vi "Main_UI.vi"(0 "Wait_Time (sec)":i32=2 caption="Wait Time (sec)" min=2, 5 "Exit":bool, 7 "Error_Log":bool caption="Error Log") -> (3 "BI_Error":T2 caption="Error?", 4 "Last_Read_PSRR (dB)":i32 caption="Last Read PSRR (dB)", 6 "Last_Error_Details":T1 caption="Last Error Details", 8 "Obtained_PSRR":i32(graph) caption="Obtained PSRR", 10 "Error_Log_Table":string[][](table) caption="Error Log Table")   [LabVIEW 2021]
doc: "This is the Main UI that Interact With the User"
uses:
  Controls/Update_Event.ctl
  Controls/Last_Error_Details.ctl
  Controls/BI_Error.ctl
panel:
  out "Error_Out":errorcluster
  in  "Error_In":errorcluster
  # "PSRR Monitor"
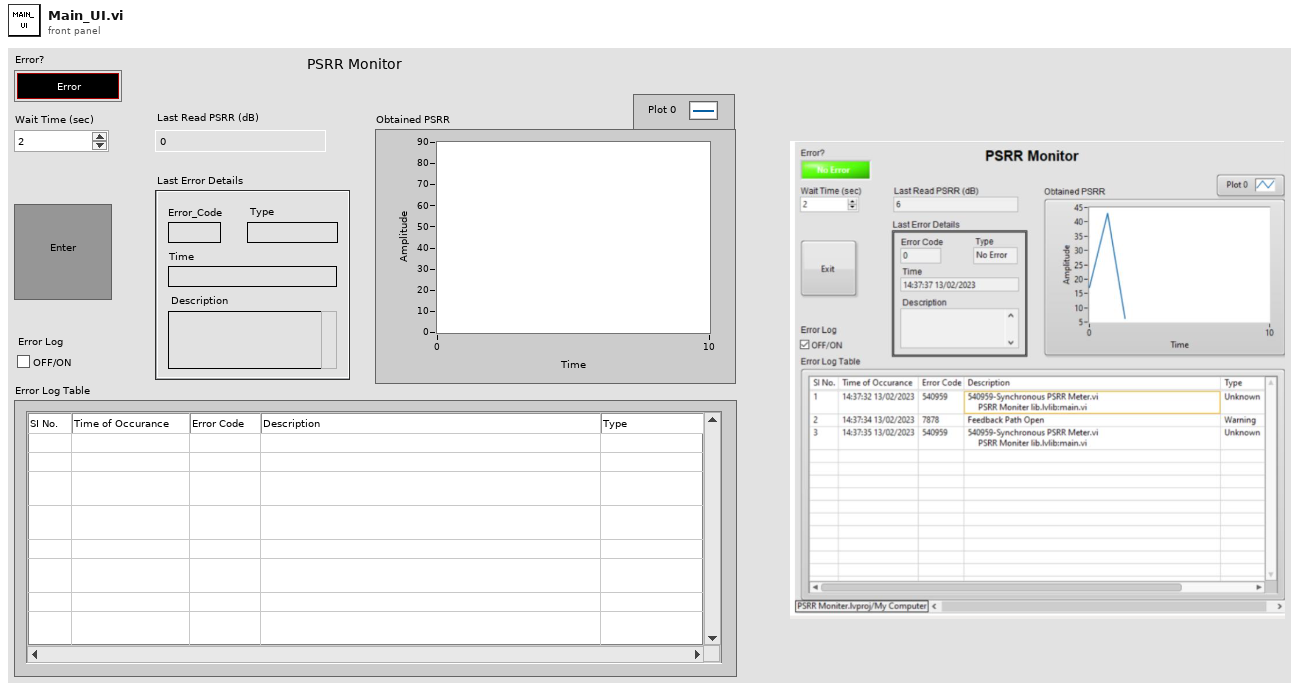
[diagram p1: front panel]
types:
  T1 = typedef "Last_Error_Details.ctl" = cluster{"Error_Code":string, "Type":string, "Time":string, "Description":string}
  T2 = typedef "BI_Error.ctl" = bool
  T3 = typedef "Update_Event.ctl" = cluster{"Exit":bool, "Wait_Time (sec)":i32}
  T4 = typedef "Obtained_PSRR_Data.ctl" = cluster{"Data":i32, "Obtained_PSRR_Data_Operation":T5}
  T5 = typedef "Obtained_PSRR_Data_Operation.ctl" = enum16{"Update", "Dont_Update", "Clear"}
  T6 = typedef "BI_Error_Con.ctl" = cluster{"Error?_Color":cluster{u32, u32}[], "Error?_Text":string}
  T7 = enum16{"Left Button", "Center Button", "Right Button", "Window Close"}
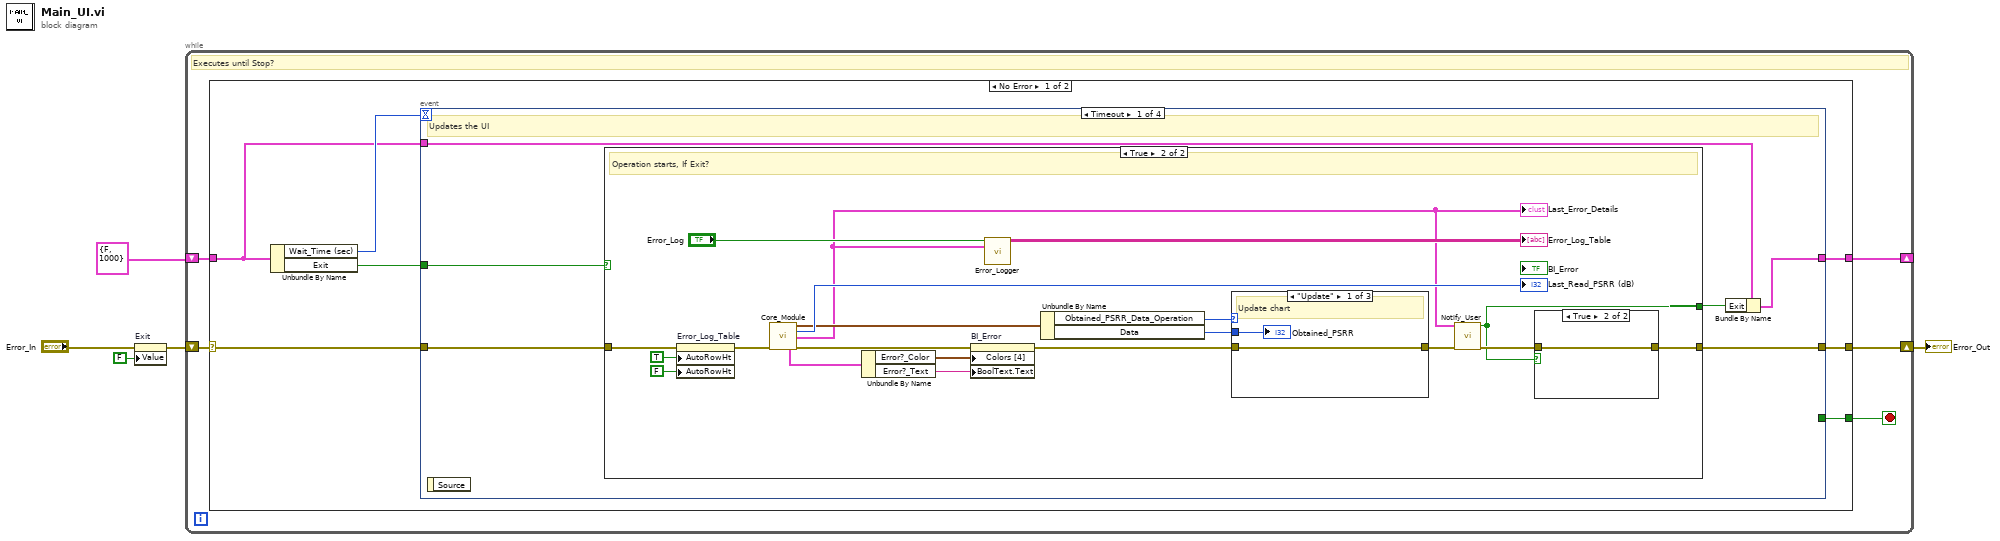
[diagram p0: block diagram]
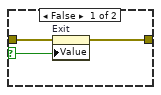
[diagram p3: hidden frame]
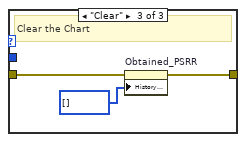
[diagram p5: hidden frame]
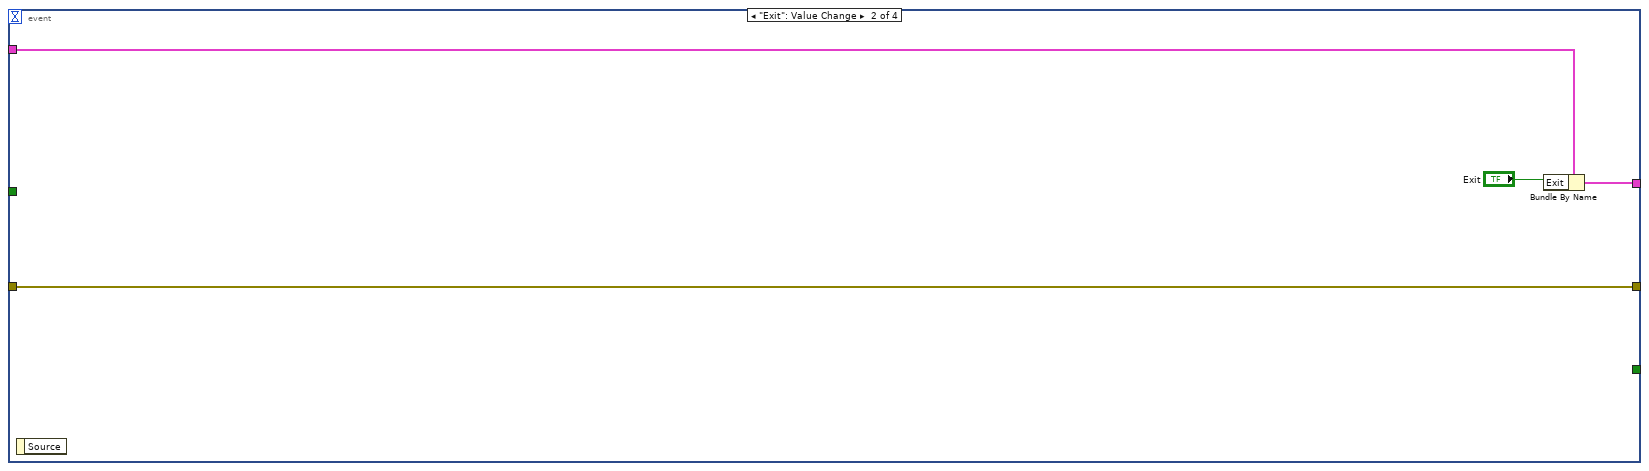
[diagram p6: hidden frame]
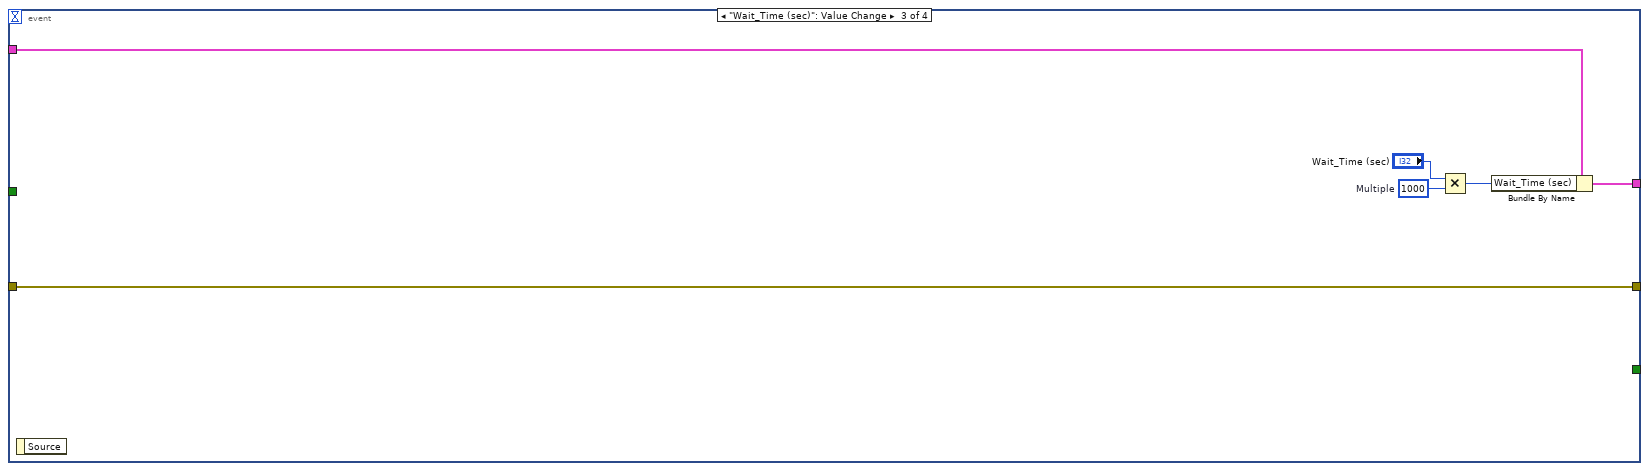
[diagram p7: hidden frame]
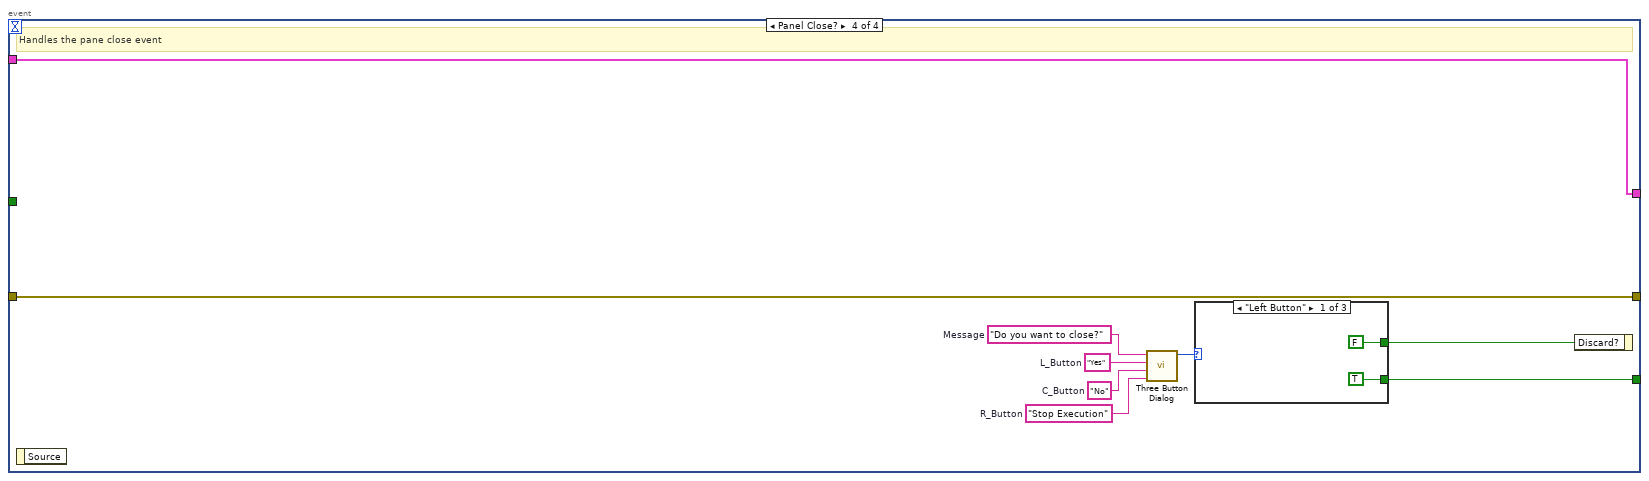
[diagram p8: hidden frame]
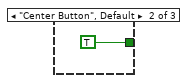
[diagram p9: hidden frame]
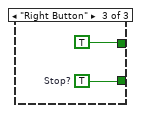
[diagram p10: hidden frame]
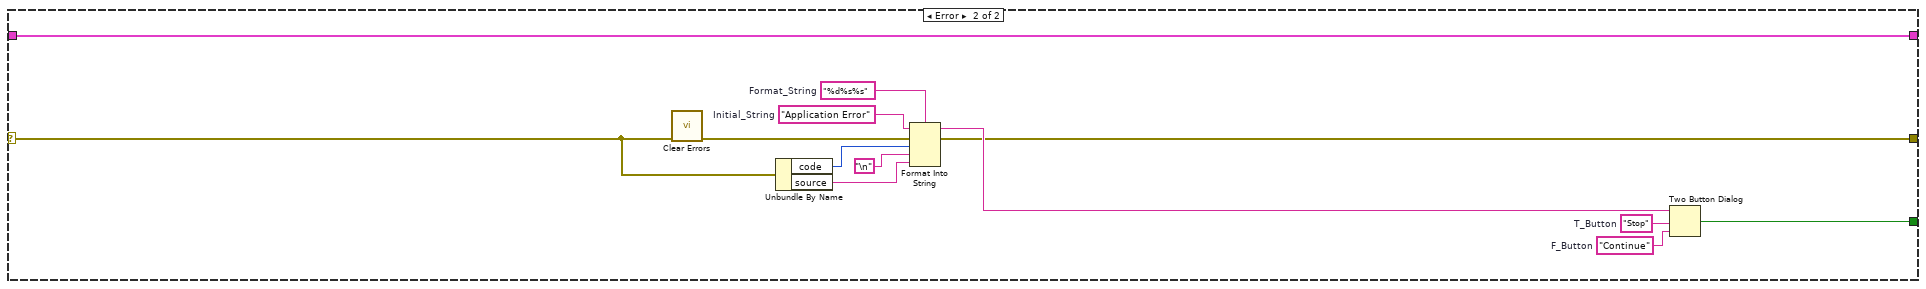
[diagram p11: hidden frame]
diagram:
  n1 = property on="Exit" class="Bool (strict)"(error in="Error_In", "Value"=FALSE ("Exit")) -> (error out=w1:errorcluster)  [unwired: 1 in, 1 out]
  n2 = while {
    shift-right: [w10] -> w5
    shift-left: w1 -> [w8]
    shift-right: [w6] -> _
    shift-left: T3 {"Exit"=FALSE, "Wait_Time (sec)"=1000} -> [w7]
    stop <- w9 stop-if-true
    # "Executes until Stop?"
    n3 = case shown="No Error" w8 {
      selector: w8 -> [w17 w83]
      tunnel: [w16 w82] -> w10
      tunnel: [w15 w81] -> w9
      tunnel: w7 -> [w12 w80]
      tunnel: [w11 w80] -> w6
      frame No Error {
        n4 = Unbundle By Name(w12) -> ("Wait_Time (sec)"=w14:i32, "Exit"=w13:bool)
        n5 = event shown="[0] Timeout" {
          selector: _ -> [_ _ _ _]
          dyn-events: _ -> [_ _ _ _]
          timeout: w14 -> [_ _ _ _]
          tunnel: w17 -> [w22 w56 w63 w67]
          tunnel: [w23 w56 w63 w67] -> w16
          tunnel: [_ _ _ w69] -> w15
          tunnel: w13 -> [w21 _ _ _]
          tunnel: w12 -> [w20 w59 w65 w66]
          tunnel: [w18 w57 w64 w66] -> w11
          event Timeout {
            # "Updates the UI"
            n6 = event-data() -> ()  [unwired: 1 in, 1 out]
            n7 = case shown="True" w21 {
              selector: w21 -> [w24 _]
              tunnel: w22 -> [w25 w28]
              tunnel: [w25 w27] -> w23
              tunnel: [w24 w26] -> w19
              frame False {
              }
              frame True {
                # "Operation starts, If Exit?"
                n8 = property on="Error_Log_Table" class="Tbl (strict)"(error in=w28, "AutoRowHt"=TRUE ("Autosizing Row Height"), "AutoRowHt"=FALSE ("Autosizing Row Height")) -> (error out=w29:errorcluster)  [unwired: 1 in, 1 out]
                n9 = call "Core_Module.vi"("Error_In"=w29) -> ("Obtained_PSRR_Data"=w40:T4, "Last_Read_PSRR (dB)"=→"Last_Read_PSRR (dB)":i32, "Last_Error_Details"=w32:T1, "Colors [4]"=w44:T6, "Error_Out"=w45:errorcluster)  [unwired: 10 in]
                "Last_Error_Details" <- w32
                n10 = Unbundle By Name(w44) -> ("Error?_Color"=w42:cluster{u32, u32}[], "Error?_Text"=w43:string)
                n11 = property on="BI_Error" class="Bool (strict)"(error in=w45, "Colors [4]"=w42, "BoolText.Text"=w43) -> (error out=w37:errorcluster)  [unwired: 1 in, 1 out]
                n12 = call "Error_Logger.vi"("Error_Log"="Error_Log", "Last_Error_Details"=w32) -> ("Error_Log_Table"=→"Error_Log_Table":string[][])  [unwired: 13 in]
                n13 = Unbundle By Name(w40) -> ("Obtained_PSRR_Data_Operation"=w39:T5, "Data"=w38:i32)
                n14 = case shown="\"Update\"" w39 {
                  tunnel: w38 -> [w51 _ _]
                  tunnel: w37 -> [w50 w52 w54]
                  tunnel: [w50 w52 w53] -> w34
                  frame "Update" {
                    # "Update chart"
                    "Obtained_PSRR" <- w51
                  }
                  frame "Dont_Update" {
                    # "Dont Update chart"
                  }
                  frame "Clear" {
                    # "Clear the Chart"
                    n15 = property on="Obtained_PSRR" class="WFChart (strict)"(error in=w54, "History Data"=i32[] []) -> (error out=w53:errorcluster)  [unwired: 1 in, 1 out]
                  }
                }
                n16 = call "Notify_User.vi"("Last_Error_Details"=w32, "Error_In"=w34) -> ("Exit?"=w26:bool, "Error_Out"=w33:errorcluster)  [unwired: 12 in]
                n17 = case shown="True" w26 {
                  selector: w26 -> [w46 _]
                  tunnel: w33 -> [w48 w49]
                  tunnel: [w47 w49] -> w27
                  frame False {
                    n18 = property on="Exit" class="Bool (strict)"(error in=w48, "Value"=w46) -> (error out=w47:errorcluster)  [unwired: 1 in, 1 out]
                  }
                  frame True {
                  }
                }
              }
            }
            n19 = Bundle By Name(cluster=w20, "Exit"=w19) -> (w18:T3)
          }
          event "Exit": Value Change {
            n20 = event-data() -> ()  [unwired: 1 in, 1 out]
            n21 = Bundle By Name(cluster=w59, "Exit"="Exit") -> (w57:T3)
          }
          event "Wait_Time (sec)": Value Change {
            w60 = 1000  # Multiple
            n22 = event-data() -> ()  [unwired: 1 in, 1 out]
            n23 = Multiply(x="Wait_Time (sec)", y=w60) -> (x*y=w62:i32)
            n24 = Bundle By Name(cluster=w65, "Wait_Time (sec)"=w62) -> (w64:T3)
          }
          event Panel Close? {
            w71 = "Stop Execution"  # R_Button
            w72 = "No"  # C_Button
            w73 = "Yes"  # L_Button
            w74 = "Do you want to close?"  # Message
            # "Handles the pane close event"
            n25 = event-data() -> ()  [unwired: 1 in, 1 out]
            n26 = call <vilib>:"Three Button Dialog.vi"("Right Button Text (\"Cancel\")"=w71, "Center Button Text (\"No\")"=w72, "Left Button Text (\"Yes\")"=w73, "message"=w74) -> ("Which Button?"=w70:T7)  [unwired: 7 in]
            n27 = case shown="\"Left Button\"" w70 {
              tunnel: [FALSE TRUE TRUE] -> w68
              tunnel: [TRUE _ w79] -> w69
              frame "Left Button" {
              }
              frame "Center Button", Default {
              }
              frame "Right Button" {
                w79 = TRUE  # Stop?
              }
            }
            n28 = event-data("Discard?"=w68) -> ()  [unwired: 1 in, 1 out]
          }
        }
      }
      frame Error {
        w88 = "%d%s%s"  # Format_String
        w89 = "Application Error"  # Initial_String
        w90 = "Stop"  # T_Button
        w91 = "Continue"  # F_Button
        n29 = call <vilib>:"Clear Errors.vi"("error in (no error)"=w83) -> ("error out"=w86:errorcluster)  [unwired: 5 in, 1 out]
        n30 = Unbundle By Name(w83) -> ("code"=w85:i32, "source"=w84:string)
        n31 = Format Into String(format string=w88, initial string=w89, error in=w86, w85, "\n", w84) -> (resulting string=w92:string, error out=w82:errorcluster)
        n32 = Two Button Dialog(message=w92, 1:w91, 2:w90) -> (T button?=w81:bool)
      }
    }
  }
  "Error_Out" <- w5
